vi "Collect_Beam_Positions.vi"(1 "Align Probe Using":enum16{"Green Beams", "Blue Beams"}(ring), 2 "Use Specification Beam Half-Angle":bool) -> ()   [LabVIEW 2018]
uses:
  Controls/Tunnel_Coordinates.ctl
  Controls/User_Specific_mode.ctl
  Globals/Trav_pos_global.vi
  Globals/Constants_global.vi
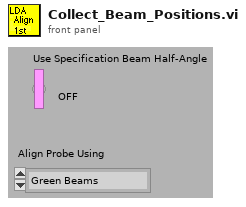
[diagram p1: front panel]
types:
  T1 = typedef "Tunnel_Coordinates.ctl" = enum16{"Work in Tunnel Coordinates", "Work in Model Coordinates"}
  T2 = typedef "User_Specific_mode.ctl" = enum16{"Check VI only", "Run VI"}
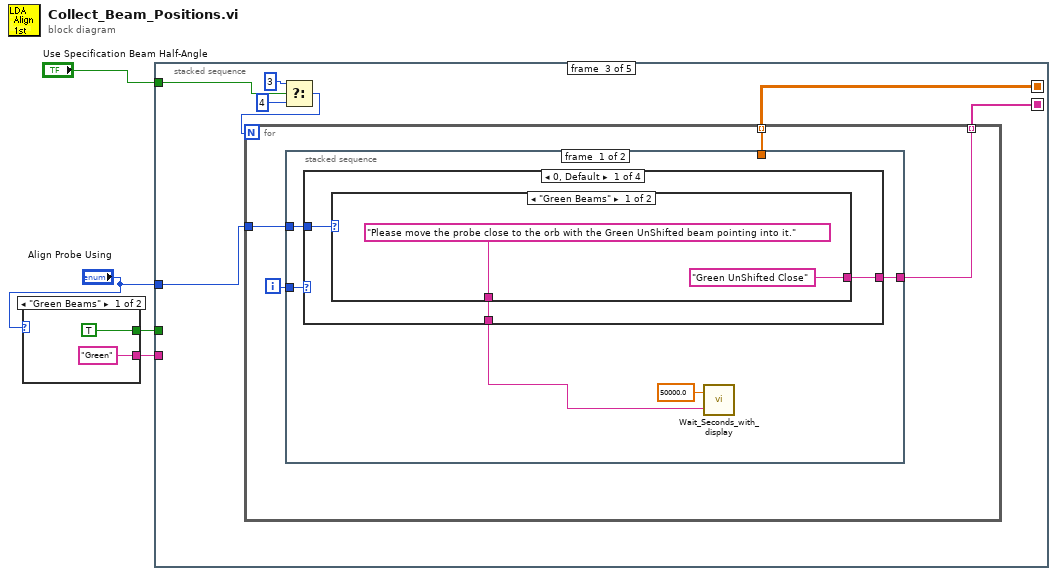
[diagram p0: block diagram]
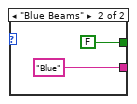
[diagram p2: hidden frame]
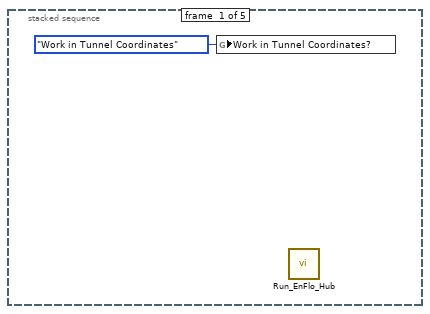
[diagram p3: hidden frame]
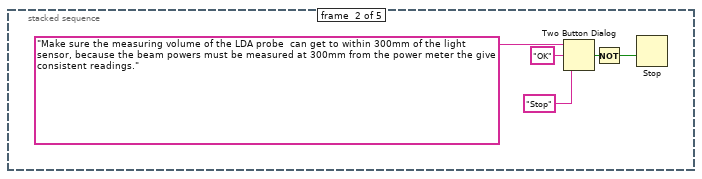
[diagram p4: hidden frame]
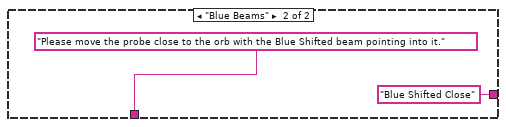
[diagram p5: hidden frame]
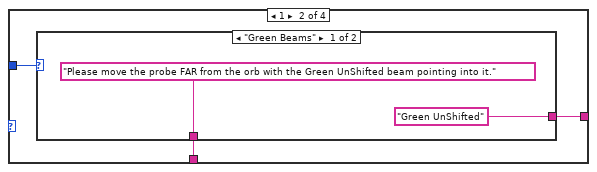
[diagram p6: hidden frame]
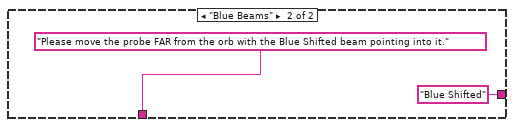
[diagram p7: hidden frame]
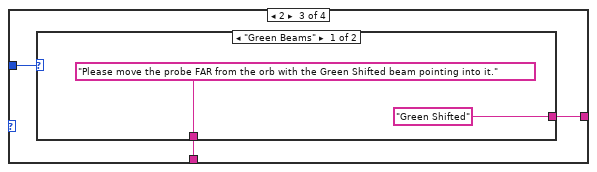
[diagram p8: hidden frame]
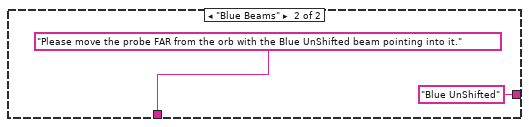
[diagram p9: hidden frame]
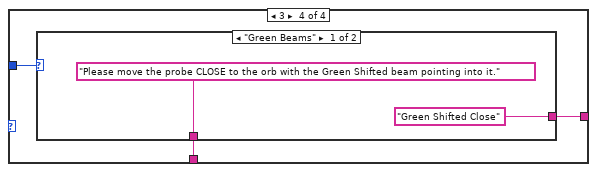
[diagram p10: hidden frame]
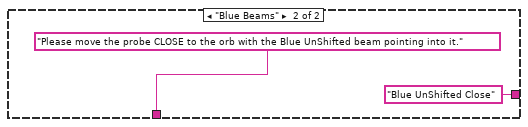
[diagram p11: hidden frame]
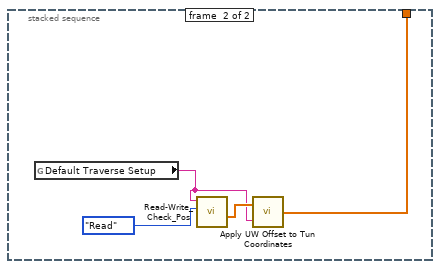
[diagram p12: hidden frame]
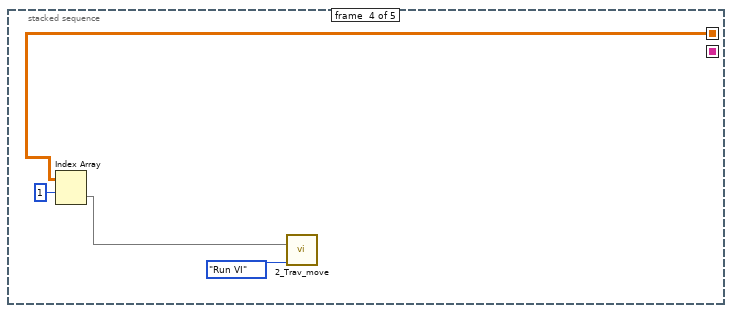
[diagram p13: hidden frame]
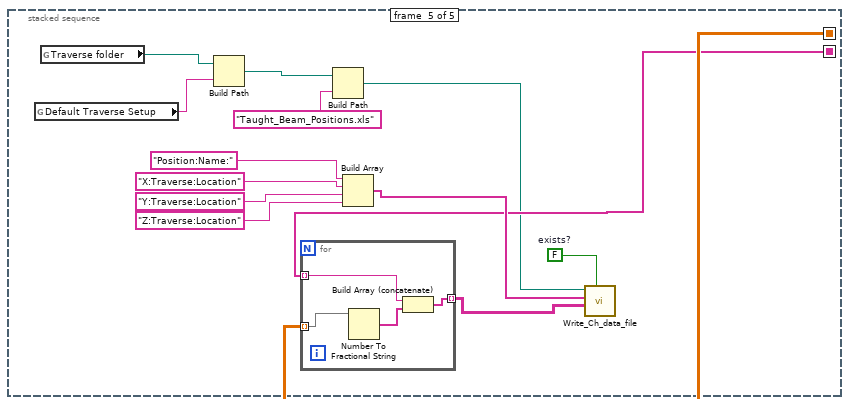
[diagram p14: hidden frame]
diagram:
  n1 = case shown="\"Green Beams\"" "Align Probe Using" {
    tunnel: [TRUE FALSE] -> w4
    tunnel: ["Green" "Blue"] -> w1
    frame "Green Beams" {
    }
    frame "Blue Beams" {
    }
  }
  n2 = stacked-sequence {
    seq-local: [_ _ w16 _ _] -> [_ _ _ w65 w70]
    seq-local: [_ _ w15 _ _] -> [_ _ _ _ w69]
    tunnel: w4 -> [_ _ _ _ _]
    tunnel: "Use Specification Beam Half-Angle" -> [_ _ w20 _ _]
    tunnel: "Align Probe Using" -> [_ _ w21 _ _]
    tunnel: w1 -> [_ _ _ _ _]
    frame #0 {
      n3 = global write "Trav_pos_global.vi" "Work in Tunnel Coordinates?"(Tunnel_Coordinates."Work in Tunnel Coordinates" ("Work in Tunnel Coordinates?")) -> ()
      n4 = call "Run_EnFlo_Hub.vi"() -> ()  [unwired: 1 in, 7 out]
    }
    frame #1 {
      n5 = Two Button Dialog(message="Make sure the measuring volume of the LDA probe  can get to within 300mm of the light sensor, because the beam powers must be measured at 300mm from the power meter the give consistent readings.", 1:"Stop" ("F button name (\"Cancel\")"), 2:"OK" ("T button name (\"OK\")")) -> (T button?=w11:bool)
      n6 = Not(x=w11) -> (.not. x?=w10:bool)
      n7 = Stop(stop? (T)=w10) -> ()
    }
    frame #2 {
      n8 = Select(t=3, s=w20, f=4) -> (s? t:f=w17:i32)
      n9 = for {
        N: w17 -> [_]
        tunnel: [w25] -> w16 mode=indexing
        tunnel: w21 -> [w24]
        tunnel: [w23] -> w15 mode=indexing
        i -> [w22]
        n10 = stacked-sequence {
          tunnel: [_ w59] -> w25
          tunnel: w24 -> [w29 _]
          tunnel: [w28 _] -> w23
          tunnel: w22 -> [w27 _]
          frame #0 {
            n11 = case shown="0, Default" w27 {
              tunnel: [w33 w40 w47 w54] -> w30
              tunnel: w29 -> [w32 w39 w46 w53]
              tunnel: [w31 w38 w45 w52] -> w28
              frame 0, Default {
                n12 = case shown="\"Green Beams\"" w32 {
                  tunnel: ["Please move the probe close to the orb with the Green UnShifted beam pointing into it." ("message") "Please move the probe close to the orb with the Blue Shifted beam pointing into it." ("message")] -> w33
                  tunnel: ["Green UnShifted Close" "Blue Shifted Close"] -> w31
                  frame "Green Beams" {
                  }
                  frame "Blue Beams" {
                  }
                }
              }
              frame 1 {
                n13 = case shown="\"Green Beams\"" w39 {
                  tunnel: ["Please move the probe FAR from the orb with the Green UnShifted beam pointing into it." ("message") "Please move the probe FAR from the orb with the Blue Shifted beam pointing into it." ("message")] -> w40
                  tunnel: ["Green UnShifted" "Blue Shifted"] -> w38
                  frame "Green Beams" {
                  }
                  frame "Blue Beams" {
                  }
                }
              }
              frame 2 {
                n14 = case shown="\"Green Beams\"" w46 {
                  tunnel: ["Please move the probe FAR from the orb with the Green Shifted beam pointing into it." ("message") "Please move the probe FAR from the orb with the Blue UnShifted beam pointing into it." ("message")] -> w47
                  tunnel: ["Green Shifted" "Blue UnShifted"] -> w45
                  frame "Green Beams" {
                  }
                  frame "Blue Beams" {
                  }
                }
              }
              frame 3 {
                n15 = case shown="\"Green Beams\"" w53 {
                  tunnel: ["Please move the probe CLOSE to the orb with the Green Shifted beam pointing into it." ("message") "Please move the probe CLOSE to the orb with the Blue UnShifted beam pointing into it." ("message")] -> w54
                  tunnel: ["Green Shifted Close" "Blue UnShifted Close"] -> w52
                  frame "Green Beams" {
                  }
                  frame "Blue Beams" {
                  }
                }
              }
            }
            n16 = call "Wait_Seconds_with_display.vi"("Message"=w30, "Seconds to wait"=50000.0) -> ()  [unwired: 1 in, 1 out]
          }
          frame #1 {
            n17 = global read "Trav_pos_global.vi" "Default Traverse Setup"() -> (w61:string)
            n18 = call "Read-Write_Check_Pos.vi"("Mode"=enum16{"Read", "Write"}."Read", "Traverse Name"=w61) -> ("Position Output"=w62:sgl[])  [unwired: 3 in, 2 out]
            n19 = call "Apply UW Offset to Tun Coordinates.vi"("Traverse Name"=w61, "Tunnel Coordinates"=w62) -> ("UW Offset Applied"=w59:sgl[])
          }
        }
      }
    }
    frame #3 {
      n20 = Index Array(array=w65, index (row)=1) -> (element=w63:sgl[])  [unwired: 1 in]
      n21 = call "2_Trav_move.vi"("New Position"=w63, "Simulate/Run"=User_Specific_mode."Run VI") -> ()  [unwired: 11 in, 3 out]
    }
    frame #4 {
      w72 = FALSE  # exists?
      n22 = global read "Trav_pos_global.vi" "Default Traverse Setup"() -> (w79:string)
      n23 = global read "Constants_global.vi" "Traverse folder"() -> (w77:path)
      n24 = Build Path(base path=w77, name or relative path=w79) -> (appended path=w78:path)
      n25 = for {
        tunnel: w70 -> [w84] mode=indexing
        tunnel: w69 -> [w83] mode=indexing
        tunnel: [w81] -> w68 mode=indexing
        n26 = Number To Fractional String(number=w84) -> (F-format string=w82:string[])  [unwired: 3 out]
        n27 = Build Array (concatenate)(w83, w82) -> (w81:string[])
      }
      n28 = Build Path(base path=w78, name or relative path="Taught_Beam_Positions.xls" ("Substring")) -> (appended path=w67:path)
      n29 = Build Array("Position:Name:", "X:Traverse:Location", "Y:Traverse:Location", "Z:Traverse:Location") -> (w71:string[])
      n30 = call "Write_Ch_data_file.vi"("exists?"=w72, "Channel Values"=w68, "Channel names"=w71, "Filename"=w67) -> ()  [unwired: 3 in, 5 out]
    }
  }
